vi "FRCts20_Backend_Stats_Reform_EventSW.vi"(8 "Error In":errorcluster, 11 "data":T1(array[cluster])) -> (0 "Error Out":errorcluster, 3 "Array":T2(array[cluster]))   [LabVIEW 2014, in "FRCts20_Backend_Engine.lvlib"]
uses:
  FRCts20_Backend_Engine.lvlib
  FRCts20_Backend_API/FRCts20_Backend_API_Stats.ctl
  ESP Engine/source/VI Source/TypeDefs/FRCts20_EspEngine_RequestPerHour_Line.ctl
  ESP Engine/source/VI Source/TypeDefs/FRCts20_EspEngine_SwUsage_Pie.ctl
  ESP Engine/source/VI Source/TypeDefs/FRCts20_EspEngine_AdvancedComponents_Bar.ctl
  ESP Engine/source/VI Source/FRCts20_EspEngine.lvlib
  FRCts20_Backend_API/FRCts20_Backend_API.lvlib
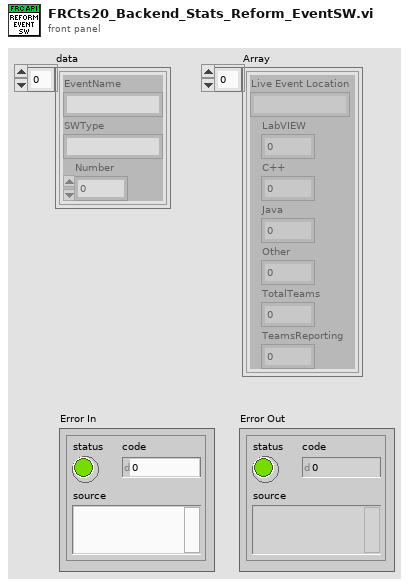
[diagram p1: front panel]
types:
  T1 = cluster{"EventName":string, "SWType":string, "Number":dbl}[]
  T2 = cluster{"Live Event Location":string, "LabVIEW":dbl, "C++":dbl, "Java":dbl, "Other":dbl, "TotalTeams":i32, "TeamsReporting":i32}[]
  T3 = typedef "FRCts20_Backend_API.lvlib/FRCts20_Backend_API_Stats.ctl" = cluster{"RequestsPerHour":T4, "SW Usage Pies":T5, "Advanced Components":T6, "APIReturn":string}
  T4 = typedef "FRCts20_EspEngine.lvlib/FRCts20_EspEngine_RequestPerHour_Line.ctl" = cluster{"StartDate":cluster{"Year":i32, "Month":i32, "Day":i32}, "Events":cluster{"Location":string, "Requests":i32[]}[]}
  T5 = typedef "FRCts20_EspEngine.lvlib/FRCts20_EspEngine_SwUsage_Pie.ctl" = cluster{"Live Event Location":string, "LabVIEW":dbl, "C++":dbl, "Java":dbl, "Other":dbl, "TotalTeams":i32, "TeamsReporting":i32}[]
  T6 = typedef "FRCts20_EspEngine.lvlib/FRCts20_EspEngine_AdvancedComponents_Bar.ctl" = cluster{"CAN":i32, "Vision":i32, "Kinect":i32}
  T7 = cluster{"Live Event Location":string, "LabVIEW":dbl, "C++":dbl, "Java":dbl, "Other":dbl, "TotalTeams":i32, "TeamsReporting":i32}
  T8 = cluster{"EventName":string, "SWType":string, "Number":dbl}
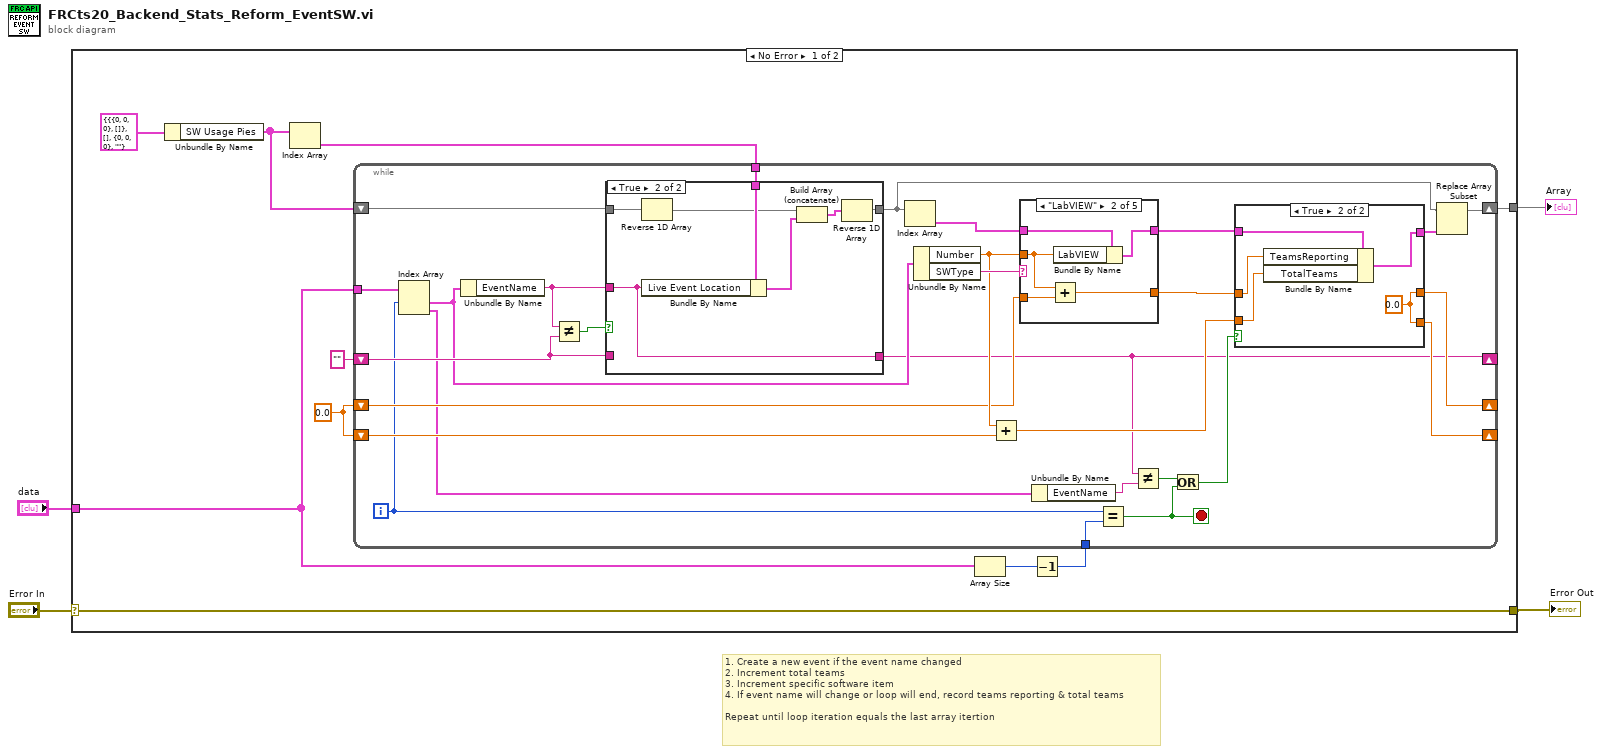
[diagram p0: block diagram]
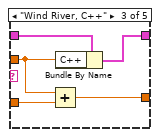
[diagram p5: hidden frame]
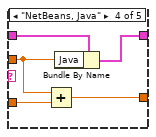
[diagram p6: hidden frame]
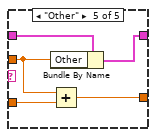
[diagram p7: hidden frame]
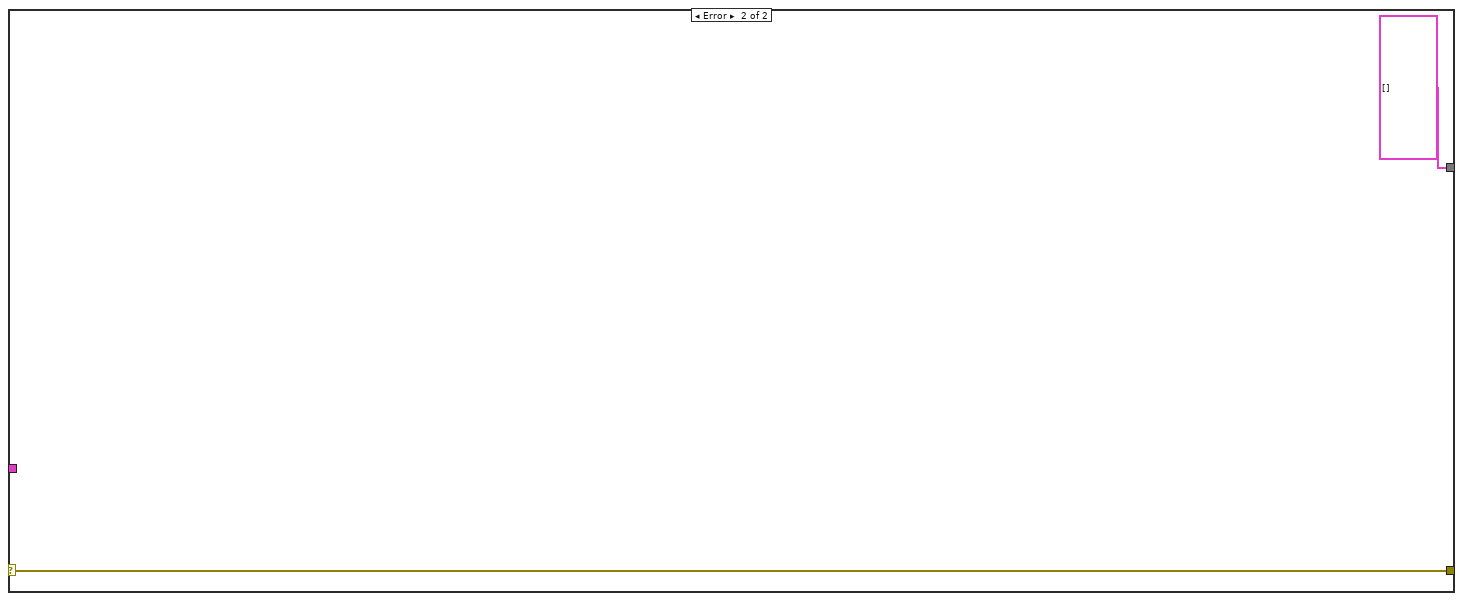
[diagram p8: hidden frame]
diagram:
  # "1. Create a new event if the event name changed\n2. Increment total teams\n3. Increment specific software item\n4. If event name will change or loop will end, record teams reporting & total teams\n\nRepeat until loop iteration equals the last array itertion"
  n1 = case shown="No Error" "Error In" {
    selector: "Error In" -> [w9 w83]
    tunnel: [w5 T2 []] -> w4
    tunnel: "data" -> [w8 _]
    tunnel: [w9 w83] -> w1
    frame No Error {
      w11 = 0.0 ("Number")
      n2 = Unbundle By Name(T3 {"RequestsPerHour"={"StartDate"={"Year"=0, "Month"=0, "Day"=0}, "Events"=[]}, "SW Usage Pies"=[], "Advanced Components"={"CAN"=0, "Vision"=0, "Kinect"=0}, "APIReturn"=""} ("Statistics")) -> ("SW Usage Pies"=w7:T5)
      n3 = Index Array(array=w7) -> (element=w6:T7)  [unwired: 1 in]
      n4 = Array Size(array=w8) -> (size(s)=w13:i32)
      n5 = Decrement(x=w13) -> (x-1=w14:i32)
      n6 = while {
        shift-right: [w40] -> _
        shift-left: w11 -> [w32]
        shift-right: [w39] -> _
        shift-left: w11 -> [w33]
        shift-right: [w16] -> _
        shift-left: "" ("EventName") -> [w35]
        tunnel: w14 -> [w27]
        tunnel: w8 -> [w20]
        shift-right: [w23] -> w5
        shift-left: w7 -> [w38]
        tunnel: w6 -> [w37]
        i -> [w19]
        stop <- w22 stop-if-true
        n7 = Index Array(array=w20, index #1=w19) -> (element #1=w21:T8, element #2=w18:T8)  [unwired: 1 in]
        n8 = Unbundle By Name(w21) -> ("EventName"=w36:string)
        n9 = Not Equal?(x=w36, y=w35) -> (x != y?=w26:bool)
        n10 = case shown="True" w26 {
          tunnel: w38 -> [w44 w51]
          tunnel: w37 -> [_ w50]
          tunnel: w36 -> [_ w49]
          tunnel: [w44 w45] -> w24
          tunnel: [w43 w49] -> w16
          tunnel: w35 -> [w43 _]
          frame False {
          }
          frame True {
            n11 = Reverse 1D Array(array=w51) -> (reversed array=w48:T5)
            n12 = Bundle By Name(cluster=w50, "Live Event Location"=w49) -> (w47:T7)
            n13 = Build Array (concatenate)(w48, w47) -> (w46:T5)
            n14 = Reverse 1D Array(array=w46) -> (reversed array=w45:T5)
          }
        }
        n15 = Index Array(array=w24) -> (element=w34:T7)  [unwired: 1 in]
        n16 = Unbundle By Name(w21) -> ("Number"=w41:dbl, "SWType"=w42:string)
        n17 = Add(x=w41, y=w33) -> (x+y=w29:dbl)
        n18 = case shown="\"LabVIEW\"" w42 {
          tunnel: [w60 w66 w71 w76 w81] -> w31
          tunnel: w41 -> [_ w65 w70 w75 w80]
          tunnel: [w61 w64 w69 w74 w79] -> w30
          tunnel: w34 -> [w60 w63 w68 w73 w78]
          tunnel: w32 -> [w61 w62 w67 w72 w77]
          frame "unknown", Default {
          }
          frame "LabVIEW" {
            n19 = Add(x=w65, y=w62) -> (x+y=w64:dbl)
            n20 = Bundle By Name(cluster=w63, "LabVIEW"=w65) -> (w66:T7)
          }
          frame "Wind River, C++" {
            n21 = Add(x=w70, y=w67) -> (x+y=w69:dbl)
            n22 = Bundle By Name(cluster=w68, "C++"=w70) -> (w71:T7)
          }
          frame "NetBeans, Java" {
            n23 = Add(x=w75, y=w72) -> (x+y=w74:dbl)
            n24 = Bundle By Name(cluster=w73, "Java"=w75) -> (w76:T7)
          }
          frame "Other" {
            n25 = Bundle By Name(cluster=w78, "Other"=w80) -> (w81:T7)
            n26 = Add(x=w80, y=w77) -> (x+y=w79:dbl)
          }
        }
        n27 = Unbundle By Name(w18) -> ("EventName"=w17:string)
        n28 = Equal?(x=w19, y=w27) -> (x = y?=w22:bool)
        n29 = Not Equal?(x=w16, y=w17) -> (x != y?=w15:bool)
        n30 = Or(x=w15, y=w22) -> (x .or. y?=w25:bool)
        n31 = case shown="True" w25 {
          tunnel: [w52 w59] -> w28
          tunnel: [w54 w58] -> w40
          tunnel: [w53 w58] -> w39
          tunnel: w31 -> [w52 w56]
          tunnel: w30 -> [w54 w57]
          tunnel: w29 -> [w53 w55]
          frame False {
          }
          frame True {
            w58 = 0.0 ("Number")
            n32 = Bundle By Name(cluster=w56, "TeamsReporting"=w57, "TotalTeams"=w55) -> (w59:T7)
          }
        }
        n33 = Replace Array Subset(array=w24, new element=w28) -> (w23:T5)  [unwired: 1 in]
      }
    }
    frame Error {
    }
  }
  "Array" <- w4
  "Error Out" <- w1
